vi "Write Time Stamp.vi"(10 "timestamp":timestamp, 11 "Properties in":refnum<class "Properties.lvclass">) -> (3 "Properties out":refnum<class "Properties.lvclass">)   [LabVIEW 2013, in "Caraya.lvlib" / "Properties.lvclass"]
uses:
  Properties.lvclass
  Properties.lvclass/Properties.ctl
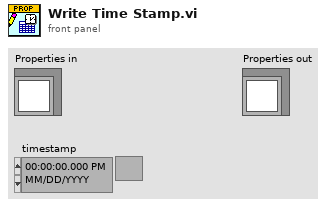
[diagram p1: front panel]
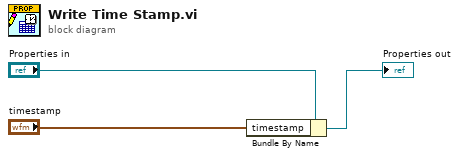
[diagram p0: block diagram]
diagram:
  n1 = Bundle By Name(cluster="Properties in", "timestamp"="timestamp") -> (→"Properties out":refnum<class "Properties.lvclass">)
